vi "18.04.2025 class.vi"() -> ()   [LabVIEW 2020]
panel:
  out "size(s)":i32
  in  "Array 2":dbl[](array[numeric])
  in  "Numeric":dbl
  out "Array":dbl[][](array[numeric])
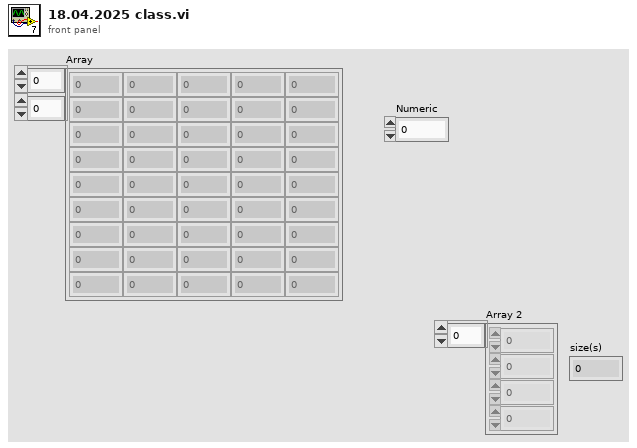
[diagram p1: front panel]
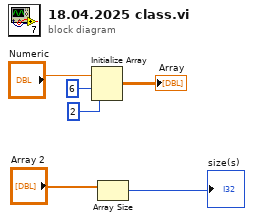
[diagram p0: block diagram]
diagram:
  n1 = Initialize Array "Initialize Array"("Numeric", 6 ("dimension size"), 2 ("dimension size")) -> (→"Array":dbl[][])
  n2 = Array Size(array="Array 2") -> (size(s)=→"size(s)":i32)
